vi "getContrastInPermille.vi"(0 "connection ID":refnum<k5>, 1 "axis":i32, 5 "error":errorcluster) -> (14 "connection ID out":refnum<k5>, 15 "axis_out":i32, 16 "contrast":i32, 17 "baseline":i32, 18 "mixcontrast":i32, 19 "error out":errorcluster)   [LabVIEW 2016, in "sen_api.lvlib"]
doc: "This function can be used to monitor the alignment contrast (peak-to-peak of the basic interference signal amplitude) and the baseline (its offset) during alignment mode."
uses:
  sen_api.lvlib
panel:
  out "jsonRespIn":string
  out "JSON-response":string="{\"jsonrpc\":\"2.0\",\"method\":\"\",\"params\":[5,1.245,true,\"name\"],\"id\":\"1\"}"
  out "JSON request":string
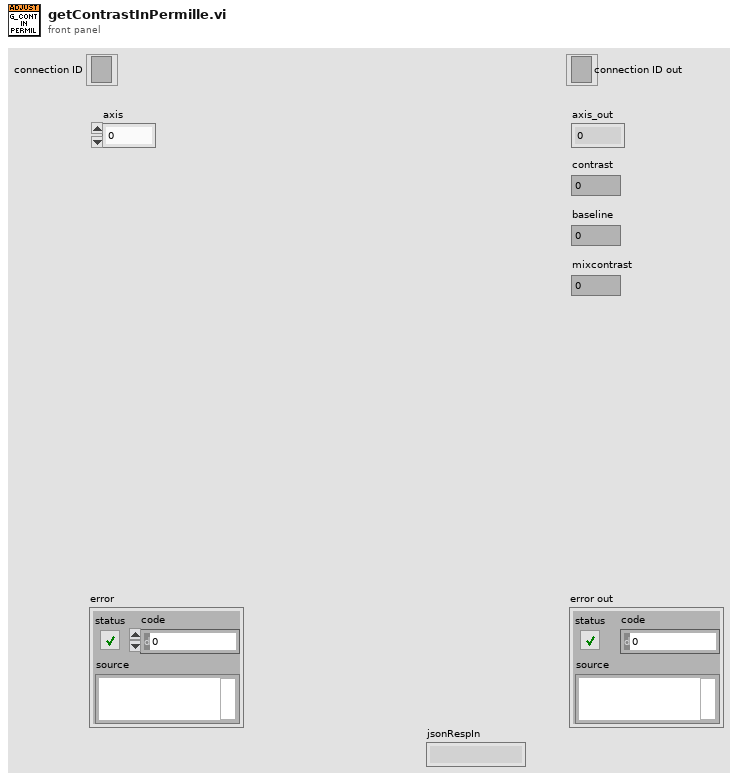
[diagram p1: front panel]
types:
  T1 = cluster{"jsonrpc":string, "method":string, "params":string[], "id":string, "api":i32, "pid":string}
  T2 = enum16{"Standard", "Buffered", "CRLF", "Immediate"}
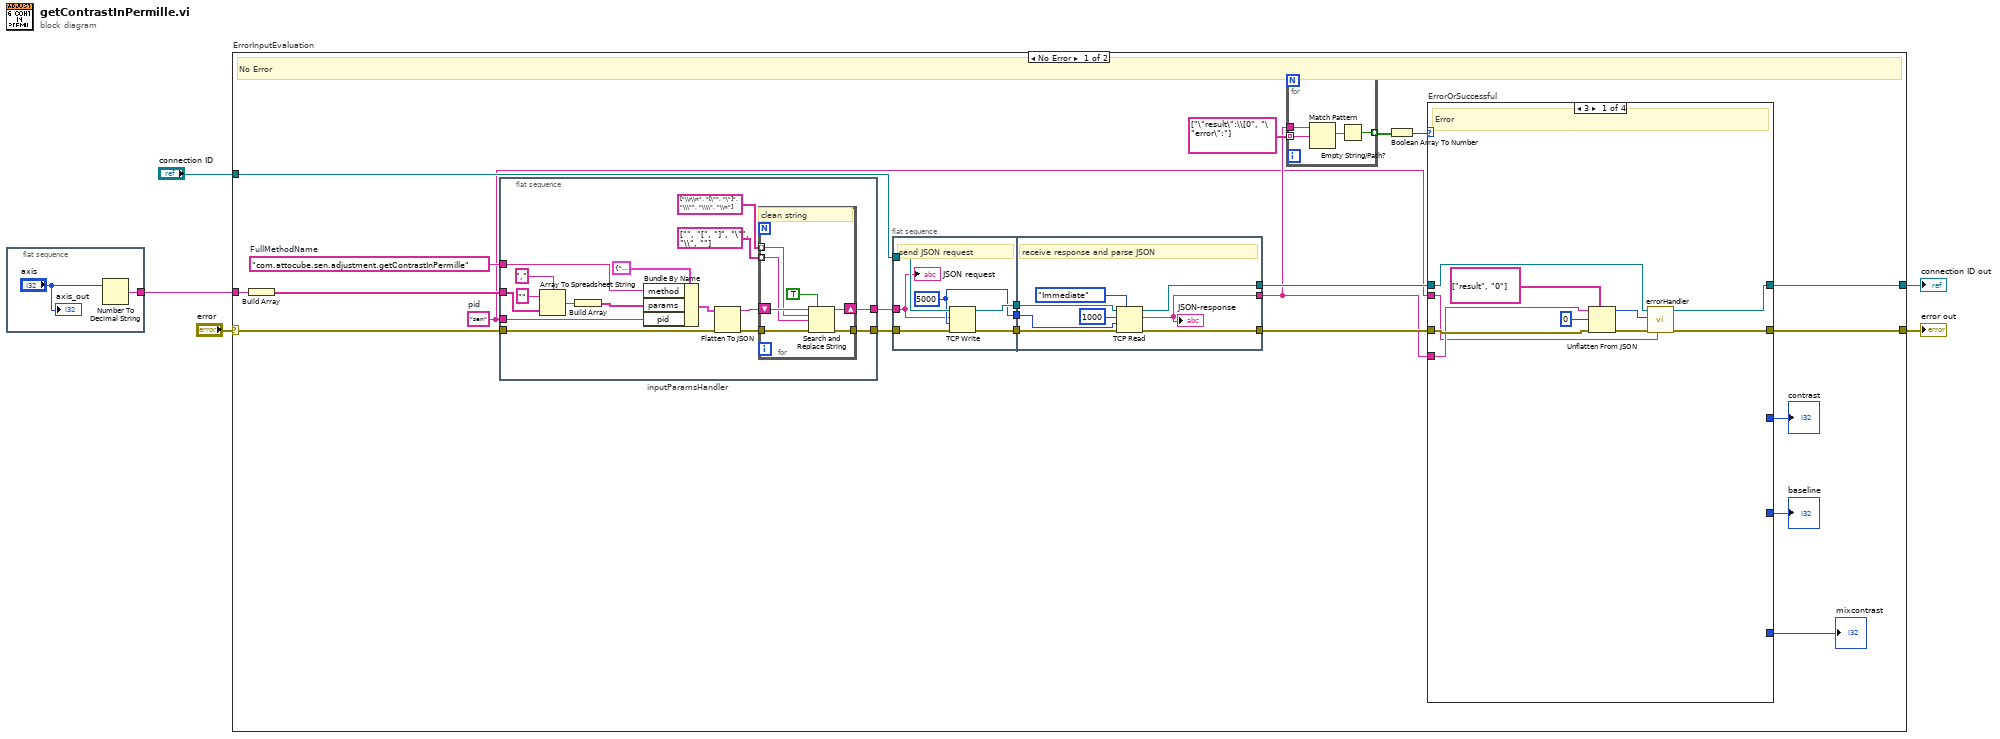
[diagram p0: block diagram]
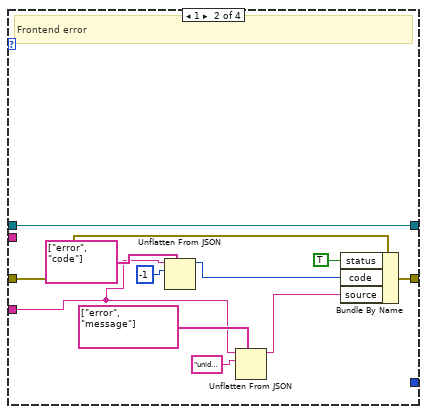
[diagram p2: hidden frame]
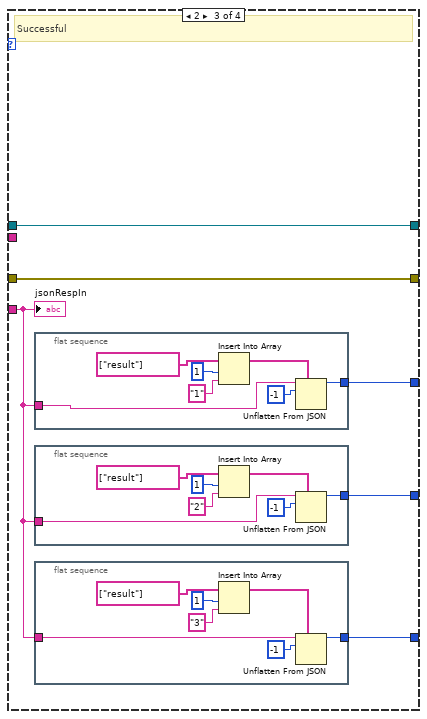
[diagram p3: hidden frame]
diagram:
  n1 = flat-sequence "in_axis" {
    tunnel: [w7] -> w1
    frame #0 {
      n2 = Number To Decimal String(number="axis") -> (decimal integer string=w7:string)  [unwired: 1 in]
      "axis_out" <- "axis"
    }
  }
  n3 = case "ErrorInputEvaluation" shown="No Error" "error" {
    selector: "error" -> [w22 w121]
    tunnel: "connection ID" -> [w26 w122]
    tunnel: [w13 w121] -> w4
    tunnel: [w14 w122] -> w3
    tunnel: w1 -> [w11 _]
    frame No Error {
      w12 = "sen"  # pid
      w23 = "com.attocube.sen.adjustment.getContrastInPermille"  # FullMethodName
      # "No Error"
      n4 = Build Array ("ParametersArrayString")(w11) -> (w21:string[])
      n5 = flat-sequence "inputParamsHandler" {
        tunnel: [w83] -> w20
        tunnel: w21 -> [w90]
        tunnel: w22 -> [w88]
        tunnel: [w85] -> w19
        tunnel: w23 -> [w91]
        tunnel: w12 -> [w80]
        frame #0 {
          n6 = Array To Spreadsheet String(delimiter (Tab)=",", array=w90, 3:"" ("format string")) -> (spreadsheet string=w93:string)
          n7 = Build Array "Build Array"(w93) -> (w89:string[])
          n8 = Bundle By Name(cluster=T1 {"jsonrpc"="2.0", "method"="com.attocube.amc.res.setRESReadOutFreq", "params"=[], "id"="1", "api"=2, "pid"=""} ("Cluster"), "method"=w91, "params"=w89, "pid"=w80) -> (w92:T1)
          n9 = Flatten To JSON(anything=w92, error in (no error)=w88) -> (JSON string=w84:string, 11:w86:errorcluster)  [unwired: 1 in]
          n10 = for {
            tunnel: string[] ["\\r\\n", "[\"", "\"]", "\\\"", "\\\\", "\\n"] ("search string") -> [w99] mode=indexing
            tunnel: string[] ["", "[", "]", "\"", "\\", ""] ("replace string (\"\")") -> [w98] mode=indexing
            shift-right: [w101] -> w83
            shift-left: w84 -> [w100]
            tunnel: w86 -> [w97]
            tunnel: [w96] -> w85
            # "clean string"
            n11 = Search and Replace String(replace all?=TRUE ("replace all? (F)"), input string=w100, search string=w99, replace string=w98, error in=w97) -> (result string=w101:string, error out=w96:errorcluster)  [unwired: 3 in, 2 out]
          }
        }
      }
      n12 = flat-sequence {
        tunnel: w26 -> [w112]
        tunnel: [w110] -> w29
        tunnel: [w111] -> w28
        tunnel: w19 -> [w107]
        tunnel: [w109] -> w27
        tunnel: w20 -> [w108]
        tunnel: [w116] -> w18
        tunnel: w29 -> [w118]
        tunnel: w28 -> [w117]
        tunnel: [w114] -> w17
        tunnel: w27 -> [w115]
        tunnel: [w113] -> w16
        frame #0 {
          w109 = 5000 ("timeout ms (25000)")
          # "send JSON request"
          n13 = TCP Write(connection ID=w112, data in=w108, error in (no error)=w107, 9:w109) -> (connection ID out=w110:refnum<k5>, error out=w111:errorcluster)  [unwired: 1 out]
          "JSON request" <- w108
        }
        frame #1 {
          # "receive response and parse JSON"
          n14 = TCP Read(connection ID=w118, bytes to read=1000, error in (no error)=w117, 7:T2."Immediate" ("mode (standard)"), 9:w115) -> (connection ID out=w116:refnum<k5>, data out=w113:string, error out=w114:errorcluster)
          "JSON-response" <- w113
        }
      }
      n15 = for {
        tunnel: string[] ["\"result\":\\[0", "\"error\":"] ("path") -> [w105] mode=indexing
        tunnel: [w103] -> w24 mode=indexing
        tunnel: w16 -> [w106]
        n16 = Match Pattern(string=w106, regular expression=w105) -> (match substring=w104:string)  [unwired: 1 in, 3 out]
        n17 = Empty String/Path?(string/path=w104) -> (empty?=w103:bool)
      }
      n18 = Boolean Array To Number(Boolean array=w24) -> (number=w15:u32)
      n19 = case "ErrorOrSuccessful" shown="3" w15 {
        tunnel: w16 -> [w33 w42 w54 _]
        tunnel: w18 -> [w37 w40 w56 w79]
        tunnel: [w35 w40 w56 w79] -> w14
        tunnel: [w36 w43 w55 w78] -> w13
        tunnel: w17 -> [w39 w41 w55 w78]
        tunnel: w12 -> [w30 _ _ _]
        tunnel: [_ _ w53 _] -> w10
        tunnel: [_ _ w52 _] -> w9
        tunnel: [_ _ w51 _] -> w8
        frame 3 {
          # "Error"
          n20 = Unflatten From JSON(path=string[] ["result", "0"], JSON string=w33, type and defaults=0, error in (no error)=w39) -> (value=w31:i32, error out=w38:errorcluster)  [unwired: 3 in]
          n21 = call "errorHandler.vi"("pid"=w30, "error in"=w38, "errNbr"=w31, "connection ID"=w37) -> ("error out 2"=w36:errorcluster, "connection ID out"=w35:refnum<k5>)  [unwired: 6 in]
        }
        frame 1 {
          # "Frontend error"
          n22 = Unflatten From JSON(path=string[] ["error", "code"], JSON string=w42, type and defaults=-1) -> (value=w49:i32)  [unwired: 4 in, 1 out]
          n23 = Unflatten From JSON(path=string[] ["error", "message"], JSON string=w42, type and defaults="unidentified error") -> (value=w50:string)  [unwired: 4 in, 1 out]
          n24 = Bundle By Name(cluster=w41, "status"=TRUE, "code"=w49, "source"=w50) -> (w43:errorcluster)
        }
        frame 2 {
          # "Successful"
          n25 = flat-sequence "out_integer" {
            tunnel: w54 -> [w73]
            tunnel: [w71] -> w53
            frame #0 {
              n26 = Insert Into Array(array=string[] ["result"] ("path"), index=1, new element="1" ("idx")) -> (w75:string[])
              n27 = Unflatten From JSON(path=w75, JSON string=w73, type and defaults=-1 ("index")) -> (value=w71:i32)  [unwired: 4 in, 1 out]
            }
          }
          n28 = flat-sequence "out_integer" {
            tunnel: w54 -> [w66]
            tunnel: [w64] -> w52
            frame #0 {
              n29 = Insert Into Array(array=string[] ["result"] ("path"), index=1, new element="2" ("idx")) -> (w68:string[])
              n30 = Unflatten From JSON(path=w68, JSON string=w66, type and defaults=-1 ("index")) -> (value=w64:i32)  [unwired: 4 in, 1 out]
            }
          }
          n31 = flat-sequence "out_integer" {
            tunnel: w54 -> [w59]
            tunnel: [w57] -> w51
            frame #0 {
              n32 = Insert Into Array(array=string[] ["result"] ("path"), index=1, new element="3" ("idx")) -> (w61:string[])
              n33 = Unflatten From JSON(path=w61, JSON string=w59, type and defaults=-1 ("index")) -> (value=w57:i32)  [unwired: 4 in, 1 out]
            }
          }
          "jsonRespIn" <- w54
        }
        frame Default {
          # "NoResponse"
        }
      }
      "contrast" <- w10
      "baseline" <- w9
      "mixcontrast" <- w8
    }
    frame Error {
      # "Error"
    }
  }
  "error out" <- w4
  "connection ID out" <- w3
